vi "ITC503_Queue_commands.vi"(1 "ITC503-Control":T1={"Setpoint (K)"=0.0, "Rate (K/min)"=3.4572, "Go to Set"=FALSE, "Set Heater SP"=FALSE, "Set NV SP"=FALSE, "Change Heater Status"=FALSE, "Change NV Status"=FALSE, "Set Auto PID"=FALSE, "Stopp"=FALSE, "Control Channel"=FALSE, "Heater SP"=0.0, "NV Setpoint"=0.0} {"Rate (K/min)" format="%#4_5f"; "Setpoint (K)" format="%6_5f"}, 3 "ITC503 Queue":refnum<queue>) -> (0 "ITC503-Control New Status":T1={"Setpoint (K)"=0.0, "Rate (K/min)"=3.4572, "Go to Set"=FALSE, "Set Heater SP"=FALSE, "Set NV SP"=FALSE, "Change Heater Status"=FALSE, "Change NV Status"=FALSE, "Set Auto PID"=FALSE, "Stopp"=FALSE, "Control Channel"=FALSE, "Heater SP"=0.0, "NV Setpoint"=0.0} {"Rate (K/min)" format="%#4_5f"; "Setpoint (K)" format="%6_5f"})   [LabVIEW 2019]
uses:
  ITC503/ITC503_control.ctl
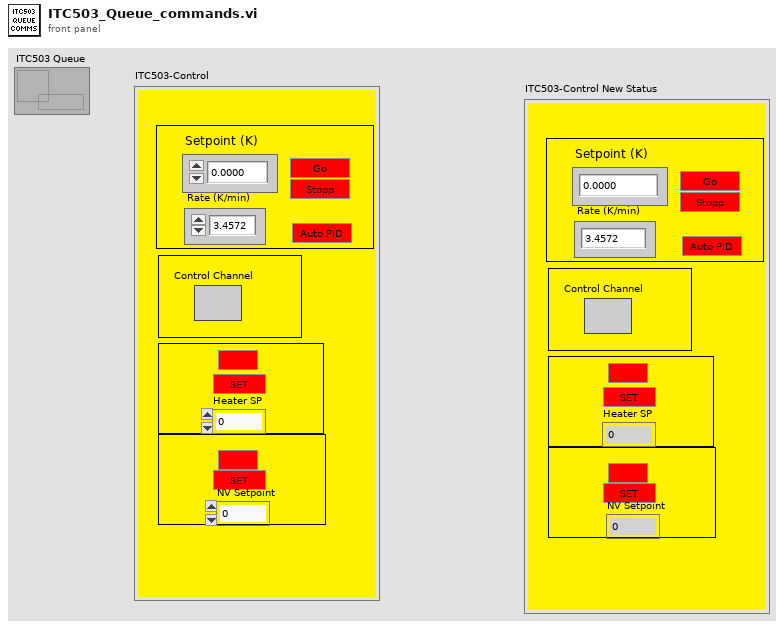
[diagram p1: front panel]
types:
  T1 = typedef "ITC503_control.ctl" = cluster{"Setpoint (K)":dbl, "Rate (K/min)":dbl, "Go to Set":bool, "Set Heater SP":bool, "Set NV SP":bool, "Change Heater Status":bool, "Change NV Status":bool, "Set Auto PID":bool, "Stopp":bool, "Control Channel":bool, "Heater SP":dbl, "NV Setpoint":dbl}
  T2 = cluster{"Setpoint (K)":bool, "Rate (K/min)":bool, "Go to Set":bool, "Set Heater SP":bool, "Set NV SP":bool, "Change Heater Status":bool, "Change NV Status":bool, "Set Auto PID":bool, "Stopp":bool, "Control Channel":bool, "Heater SP":bool, "NV Setpoint":bool}
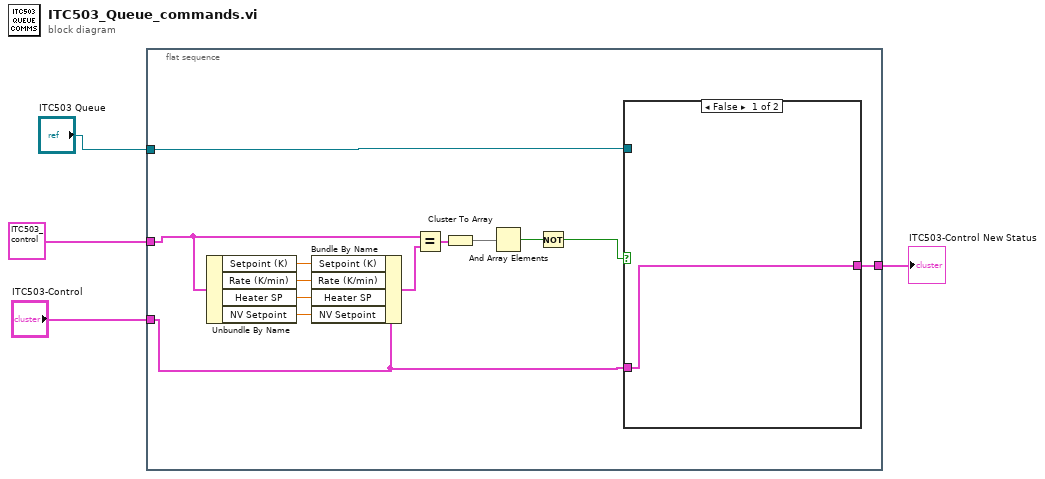
[diagram p0: block diagram]
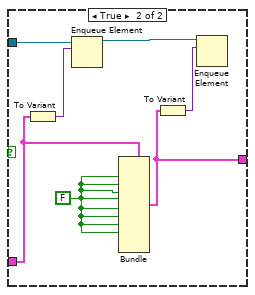
[diagram p2: hidden frame]
diagram:
  n1 = flat-sequence {
    tunnel: "ITC503 Queue" -> [w17]
    tunnel: T1 {"Setpoint (K)"=0.0, "Rate (K/min)"=3.4572, "Go to Set"=FALSE, "Set Heater SP"=FALSE, "Set NV SP"=FALSE, "Change Heater Status"=FALSE, "Change NV Status"=FALSE, "Set Auto PID"=FALSE, "Stopp"=FALSE, "Control Channel"=FALSE, "Heater SP"=0.0, "NV Setpoint"=0.0} ("ITC503-Control") -> [w16]
    tunnel: "ITC503-Control" -> [w6]
    tunnel: [w5] -> w1
    frame #0 {
      n2 = Unbundle By Name(w16) -> ("Setpoint (K)"=w14:dbl, "Rate (K/min)"=w13:dbl, "Heater SP"=w12:dbl, "NV Setpoint"=w11:dbl)
      n3 = Bundle By Name(cluster=w6, "Setpoint (K)"=w14, "Rate (K/min)"=w13, "Heater SP"=w12, "NV Setpoint"=w11) -> (w15:T1)
      n4 = Equal?(x=w16, y=w15) -> (x = y?=w10:T2)
      n5 = Cluster To Array(cluster=w10) -> (array=w9:bool[])
      n6 = And Array Elements(Boolean array=w9) -> (logical AND=w8:bool)
      n7 = Not(x=w8) -> (.not. x?=w7:bool)
      n8 = case shown="False" w7 {
        tunnel: w17 -> [_ w25]
        tunnel: w6 -> [w18 w22]
        tunnel: [w18 w19] -> w5
        frame False {
        }
        frame True {
          w21 = FALSE
          n9 = To Variant(anything=w22) -> (Variant=w23:variant)
          n10 = Enqueue Element(queue=w25, element=w23) -> (queue out=w24:refnum<queue>)  [unwired: 2 in, 2 out]
          n11 = Bundle(cluster=w22, "Go to Set"=w21, "Set Heater SP"=w21, "Set NV SP"=w21, "Change Heater Status"=w21, "Change NV Status"=w21, "Set Auto PID"=w21, "Stopp"=w21, "Control Channel"=w21) -> (w19:T1)  [unwired: 4 in]
          n12 = To Variant(anything=w19) -> (Variant=w20:variant)
          n13 = Enqueue Element(queue=w24, element=w20) -> ()  [unwired: 2 in, 3 out]
        }
      }
    }
  }
  "ITC503-Control New Status" <- w1
